vi "I-SRC Output Enable.vi"(7 "Output (Off)":bool, 8 "error in (no error)":errorcluster, 11 "VISA resource name in":refnum<visa-resource-name>) -> (0 "error out":errorcluster, 3 "VISA resource name out":refnum<visa-resource-name>)   [LabVIEW 2016, in "Hall Effect Library.lvlib"]
uses:
  Hall Effect Library.lvlib
  Global Variables/Instruments.vi
  I-SRC Output Enable (622X).vi
  I-SRC Output Enable (26XX).vi
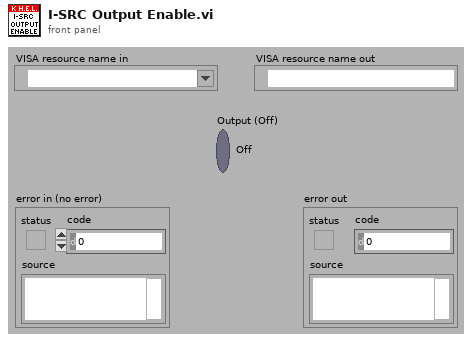
[diagram p1: front panel]
types:
  T1 = typedef "Hall Effect Library.lvlib/I-Sources.ctl" = enum16{"622X", "26XX"}
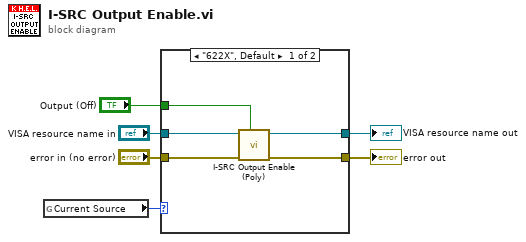
[diagram p0: block diagram]
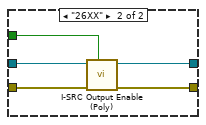
[diagram p2: hidden frame]
diagram:
  n1 = global read "Instruments.vi" "Current Source"() -> (w6:T1)
  n2 = case shown="\"622X\", Default" w6 {
    tunnel: "VISA resource name in" -> [w11 w16]
    tunnel: [w10 w15] -> w4
    tunnel: "error in (no error)" -> [w9 w14]
    tunnel: [w8 w13] -> w2
    tunnel: "Output (Off)" -> [w7 w12]
    frame "622X", Default {
      n3 = call-poly "I-SRC Output Enable (Poly).vi"("Output (Off)"=w7, "error in (no error)"=w9, "VISA resource name in"=w11) -> ("error out"=w8:errorcluster, "VISA resource name out"=w10:refnum<visa-resource-name>)  [unwired: 7 out]
    }
    frame "26XX" {
      n4 = call-poly "I-SRC Output Enable (Poly).vi"("Output (Off)"=w12, "error in (no error)"=w14, "VISA resource name in"=w16) -> ("error out"=w13:errorcluster, "VISA resource name out"=w15:refnum<visa-resource-name>)  [unwired: 7 out]
    }
  }
  "error out" <- w2
  "VISA resource name out" <- w4
